vi "GSM Sync Out.vi"(7 "Begin Timeslot (1)":i16=1, 8 "error in (no error)":errorcluster {"code" format="%.0x"}, 9 "Sync Out Offset (0)":i16, 10 "Sync Out (0:BEGIN FRAME)":T1(ring), 11 "VISA Resource Name":refnum<visa-resource-name>) -> (0 "error out":errorcluster {"code" format="%.0x"}, 3 "VISA Resource Name Out":refnum<visa-resource-name>)   [LabVIEW 2014, in "Agilent ESG Series.lvlib"]
doc: "This VI is used to configure the \"Sync Out\" parameters.\nThere is no need to run this vi if Data Format is set to Pattern because the Sync out will default to Begin Pattern."
uses:
  Agilent ESG Series.lvlib
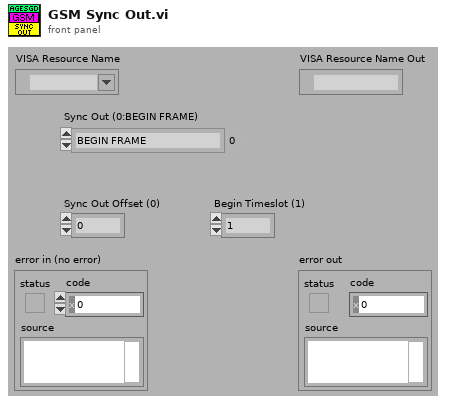
[diagram p1: front panel]
types:
  T1 = enum16{"BEGIN FRAME", "BEGIN TIMESLOT", "ALL TIMESLOTS"}
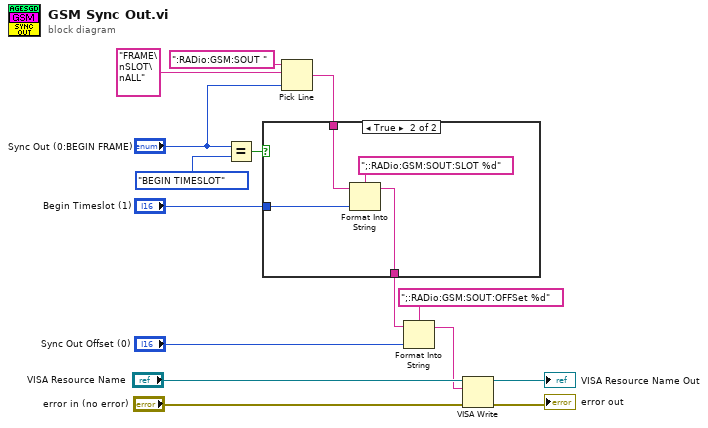
[diagram p0: block diagram]
diagram:
  n1 = Equal?(x="Sync Out (0:BEGIN FRAME)", y=T1."BEGIN TIMESLOT") -> (x = y?=w5:bool)
  n2 = Pick Line(string ("")=":RADio:GSM:SOUT ", multi-line string="FRAME\nSLOT\nALL", line index="Sync Out (0:BEGIN FRAME)") -> (output string=w9:string)
  n3 = case shown="True" w5 {
    tunnel: "Begin Timeslot (1)" -> [_ w18]
    tunnel: w9 -> [w16 w17]
    tunnel: [w16 w19] -> w4
    frame False {
    }
    frame True {
      n4 = Format Into String(format string=";:RADio:GSM:SOUT:SLOT %d", initial string=w17, w18) -> (resulting string=w19:string)  [unwired: 1 in, 1 out]
    }
  }
  n5 = Format Into String(format string=";:RADio:GSM:SOUT:OFFSet %d", initial string=w4, "Sync Out Offset (0)") -> (resulting string=w1:string)  [unwired: 1 in, 1 out]
  n6 = VISA Write(VISA resource name="VISA Resource Name", write buffer=w1, error in (no error)="error in (no error)") -> (VISA resource name out=→"VISA Resource Name Out":refnum<visa-resource-name>, error out=→"error out":errorcluster)  [unwired: 1 out]
